vi "Util_WeightedWaypoint_To_WeightedWayPoint.vi"(11 "Util_WeightedWayPoints":T4[](array[typedef]) {"WEIGHT" format="%13.3f"; "ANGLE" format="%13.3f"; "Y" format="%13.3f"; "X" format="%13.3f"}) -> (3 "WeightedWayPoints":T1[](array[typedef]) {"SCALAR" format="%14.3f"; "ROTATION"."SIN" format="%13.4f"; "ROTATION"."COS" format="%13.4f"; "ROTATION"."VALUE" format="%13.4f"; "TRANSLATION"."Y" format="%14.3f"; "TRANSLATION"."X" format="%14.3f"})   [LabVIEW 2019, in "Trajectory_Library.lvlib"]
doc: "Utility function to convert UTIL_WeightedWayPoints to WeightedWayPoints"
uses:
  Trajectory_Library.lvlib
  UTIL_WEIGHTED_WAYPOINT.ctl
  WEIGHTED_WAYPOINT.ctl
  TRANSLATION2D.ctl
  ROTATION2D.ctl
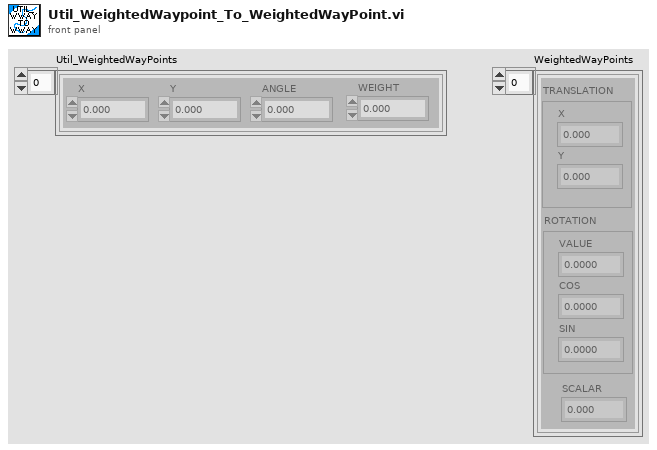
[diagram p1: front panel]
types:
  T1 = typedef "Trajectory_Library.lvlib/WEIGHTED_WAYPOINT.ctl" = cluster{"TRANSLATION":T2, "ROTATION":T3, "SCALAR":dbl}
  T2 = typedef "Trajectory_Library.lvlib/TRANSLATION2D.ctl" = cluster{"X":dbl, "Y":dbl}
  T3 = typedef "Trajectory_Library.lvlib/ROTATION2D.ctl" = cluster{"VALUE":dbl, "COS":dbl, "SIN":dbl}
  T4 = typedef "Trajectory_Library.lvlib/UTIL_WEIGHTED_WAYPOINT.ctl" = cluster{"X":dbl, "Y":dbl, "ANGLE":dbl, "WEIGHT":dbl}
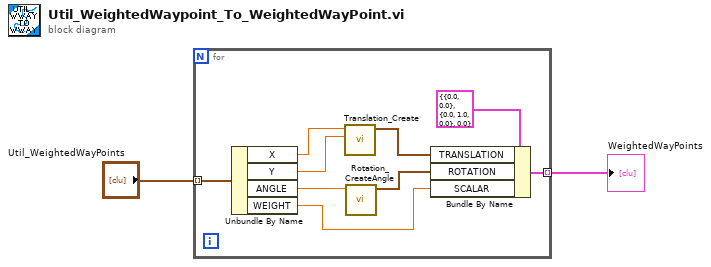
[diagram p0: block diagram]
diagram:
  n1 = for {
    tunnel: "Util_WeightedWayPoints" -> [w11] mode=indexing
    tunnel: [w3] -> w1 mode=indexing
    n2 = Unbundle By Name(w11) -> ("X"=w6:dbl, "Y"=w5:dbl, "ANGLE"=w9:dbl, "WEIGHT"=w7:dbl)
    n3 = call "Translation_Create.vi"("Y"=w5, "X"=w6) -> ("TRANSLATION"=w4:T2)  [unwired: 9 in]
    n4 = call "Rotation_CreateAngle.vi"("Angle"=w9) -> ("ROTATION"=w8:T3)  [unwired: 10 in]
    n5 = Bundle By Name(cluster=T1 {"TRANSLATION"={"X"=0.0, "Y"=0.0}, "ROTATION"={"VALUE"=0.0, "COS"=1.0, "SIN"=0.0}, "SCALAR"=0.0} ("WEIGHTED_WAYPOINT"), "TRANSLATION"=w4, "ROTATION"=w8, "SCALAR"=w7) -> (w3:T1)
  }
  "WeightedWayPoints" <- w1
